vi "经纬度及是否定位成功.vi"(11 "即时数据":string) -> (0 "纬分":dbl, 1 "纬度":i32, 2 "经分":dbl, 3 "经度":i32, 4 "定位成功":bool)   [LabVIEW 2018]
panel:
  out "航向（度）":sgl
  out "速度（节）":dbl
  out "read buffer":string
  out "RMC":bool
  out "第一个子数组":u8[](array[numeric])
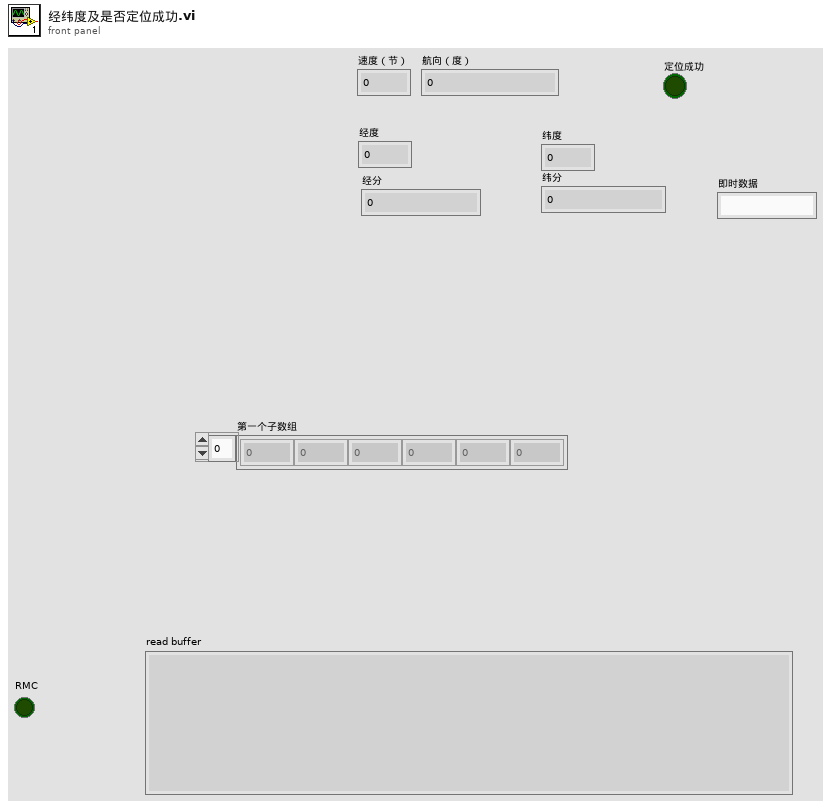
[diagram p1: front panel]
types:
  T1 = cluster{"[0]":u8, "[1]":u8, "[2]":u8, "[3]":u8, "[4]":u8, "[5]":u8, "[6]":u8, "[7]":u8, "[8]":u8}
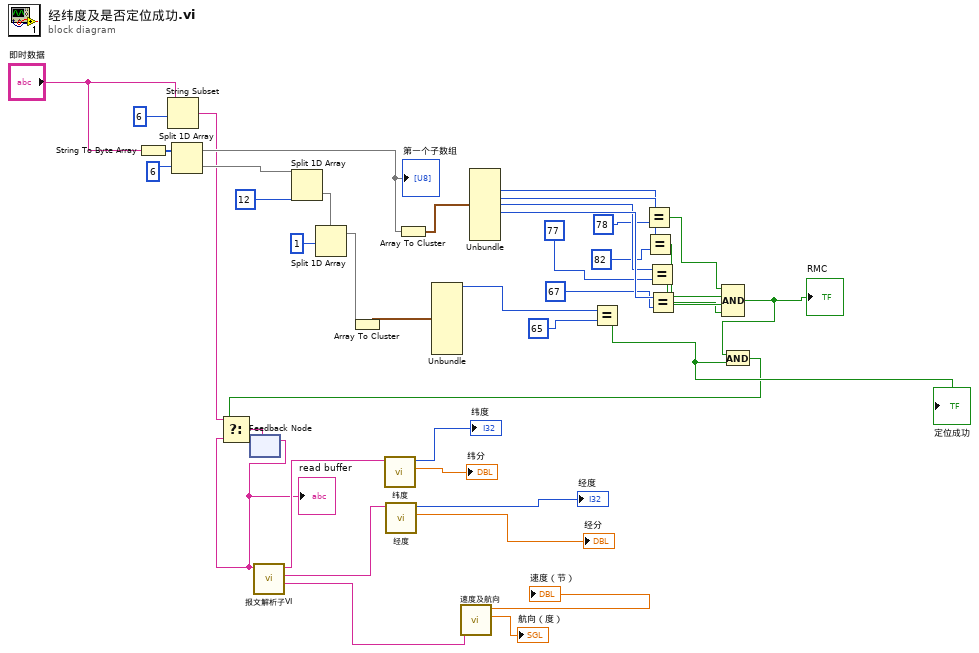
[diagram p0: block diagram]
diagram:
  n1 = String To Byte Array(string="即时数据") -> (unsigned byte array=w40:u8[])
  n2 = String Subset(string="即时数据", offset (0)=6 ("偏移量(0)")) -> (substring=w8:string)  [unwired: 1 in]
  n3 = Split 1D Array(array=w40, index=6 ("索引")) -> (first subarray=w38:u8[], second subarray=w15:u8[])
  "第一个子数组" <- w38
  n4 = feedback #1() -> (w6:string)  [unwired: 1 in]
  "read buffer" <- w6
  n5 = call "报文解析子VI.vi"("剔除报文标识字符串"=w6) -> ("速度及航向"=w12:string, "经度"=w10:string, "纬度"=w11:string)  [unwired: 6 in, 2 out]
  n6 = Split 1D Array(array=w15, index=12 ("索引")) -> (second subarray=w31:u8[])  [unwired: 1 out]
  n7 = Split 1D Array(array=w31, index=1 ("索引")) -> (first subarray=w21:u8[])  [unwired: 1 out]
  n8 = Array To Cluster(array=w21) -> (cluster=w20:T1)
  n9 = call "纬度.vi"("纬度"=w11) -> ("纬分"=→"纬分":dbl, "纬度"=→"纬度":i32)  [unwired: 8 in, 1 out]
  n10 = call "经度.vi"("经度"=w10) -> ("经分"=→"经分":dbl, "经度"=→"经度":i32)  [unwired: 8 in, 1 out]
  n11 = Array To Cluster(array=w38) -> (cluster=w37:T1)
  n12 = Unbundle(w20) -> ("[0]"=w19:u8)  [unwired: 8 out]
  n13 = call "速度及航向.vi"("速度及航向输入"=w12) -> ("航向（度）"=→"航向（度）":sgl, "速度（节）"=→"速度（节）":dbl)  [unwired: 9 in]
  n14 = Unbundle(w37) -> ("[2]"=w28:u8, "[3]"=w29:u8, "[4]"=w35:u8, "[5]"=w36:u8)  [unwired: 5 out]
  n15 = Equal?(x=w19, y=u8 65) -> (x = y?=w16:bool)
  "定位成功" <- w16
  n16 = Equal?(x=w28, y=u8 78) -> (x = y?=w25:bool)
  n17 = Equal?(x=w29, y=u8 82) -> (x = y?=w24:bool)
  n18 = Equal?(x=w35, y=u8 77) -> (x = y?=w23:bool)
  n19 = Equal?(x=w36, y=u8 67) -> (x = y?=w22:bool)
  n20 = Compound Arithmetic op=AND ("复合运算")(w25, w24, w23, w22) -> (w17:bool)
  "RMC" <- w17
  n21 = And(x=w17, y=w16) -> (x .and. y?=w9:bool)
  n22 = Select(t=w8, s=w9, f=w6) -> (s? t:f=w7:string)
  n23 = feedback-in #1(w7) -> ()
